vi "Unpack SGL Value.vi"(11 "SGLValueMsg in":refnum<class "SGLValueMsg.lvclass">) -> (2 "Value":sgl, 3 "Name":string)   [LabVIEW 2015, in "ActorAutoRegistration.lvlib" / "SGLValueMsg.lvclass"]
uses:
  SGLValueMsg.lvclass
  SGLValueMsg.lvclass/SGLValueMsg.ctl
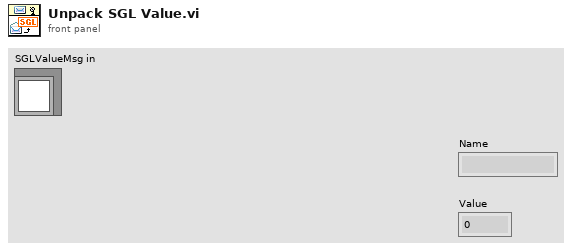
[diagram p1: front panel]
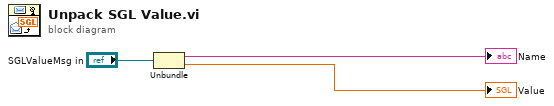
[diagram p0: block diagram]
diagram:
  n1 = Unbundle("SGLValueMsg in") -> (→"Name":string, →"Value":sgl)
